vi "Test Type Selection.vi"(0 "File Path Control":path, 11 "Error In":errorcluster) -> (3 "path":path, 4 "File Name":string, 6 "Test Type":string, 8 "Interruptions":u32, 10 "Delay":u32, 15 "Error Out":errorcluster)   [LabVIEW 2018, in "CollectionSupport.lvlib"]
uses:
  CollectionSupport.lvlib
  Controls/Mech-Labial Test Types.ctl
panel:
  in  "Sex":u16(ring) items=["Male", "Female"]
  in  "Age":string
  in  "OK Button":bool
  in  "Subject":string
  in  "Test Types":T1 items=["Practice Trials", "Mechanical (Mask)", "Mechanical (Mouthpiece)", "Labial (Normal)", "Labial (Quiet)"]
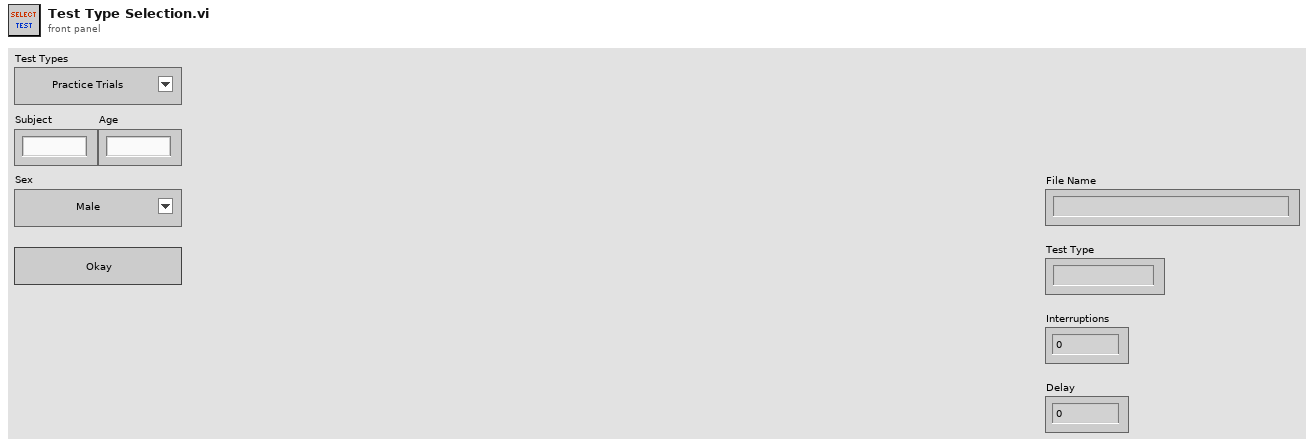
[diagram p1: front panel]
types:
  T1 = typedef "CollectionSupport.lvlib/Mech-Labial Test Types.ctl" = u16
  T2 = enum16{"open", "replace", "create", "open or create", "replace or create", "replace or create with confirmation"}
  T3 = typedef "eventvkey.ctl" = enum16{"ASCII", "Enter", "Return", "Shift", "Ctrl", "Alt", "Cmd", "Opt", "Caps", "NumLock", "Clear", "Break", "Up", "Down", "Left", "Right", "Insert", "Delete", "Home", "End", "PageUp", "PageDown", "Escape", "Help", "Pause", "ScrollLock", "F1", "F2", "F3", "F4", "F5", "F6", "F7", "F8", "F9", "F10", "F11", "F12", "F13", "F14", "F15", "F16", "F17", "F18", "F19", "F20", "F21", "F22", "F23", "F24", "Play", "VolumeUp", "VolumeDown", "Mute", "Two Byte Char"}
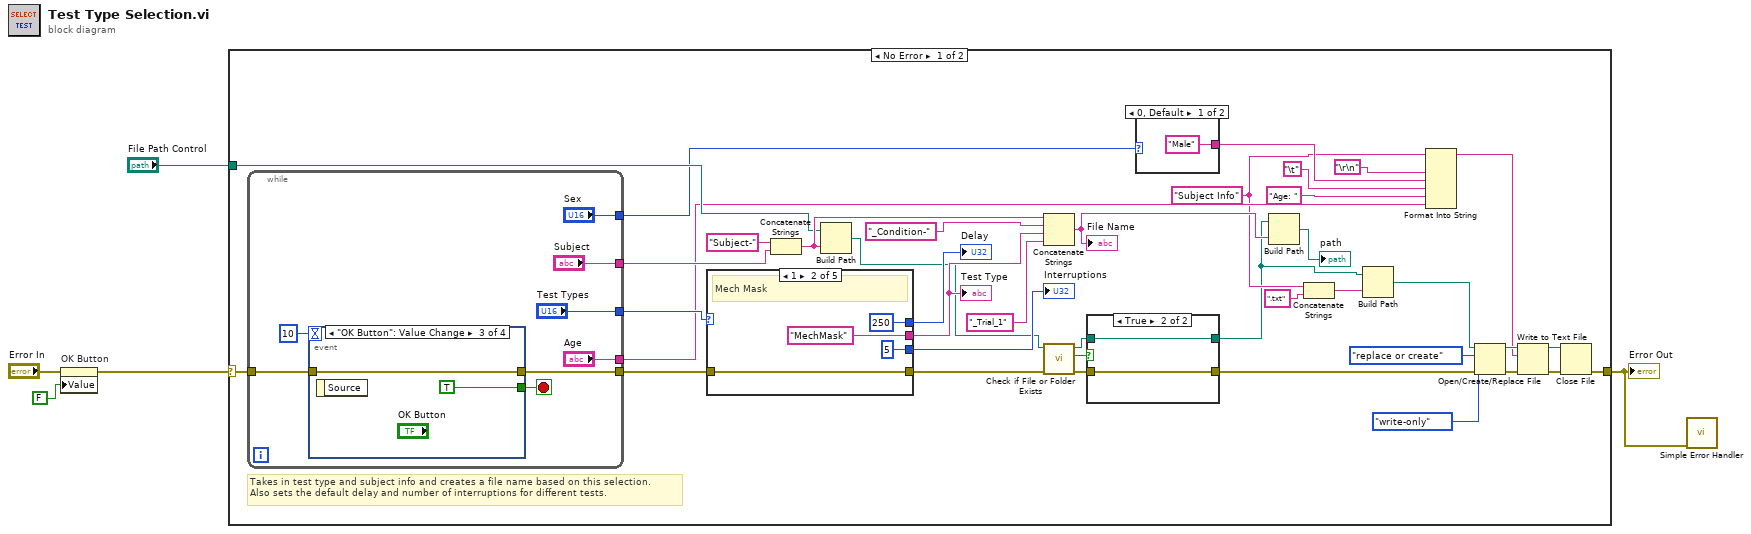
[diagram p0: block diagram]
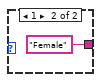
[diagram p2: hidden frame]
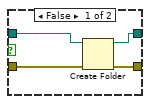
[diagram p3: hidden frame]
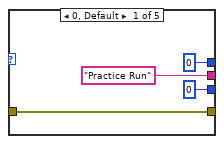
[diagram p4: hidden frame]
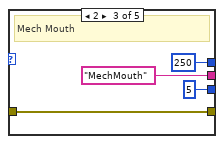
[diagram p5: hidden frame]
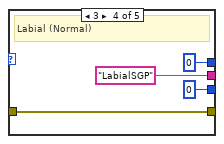
[diagram p6: hidden frame]
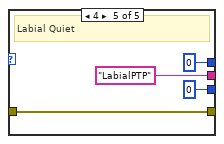
[diagram p7: hidden frame]
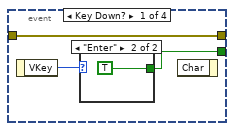
[diagram p8: hidden frame]
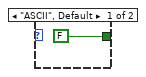
[diagram p9: hidden frame]
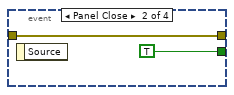
[diagram p10: hidden frame]
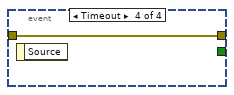
[diagram p11: hidden frame]
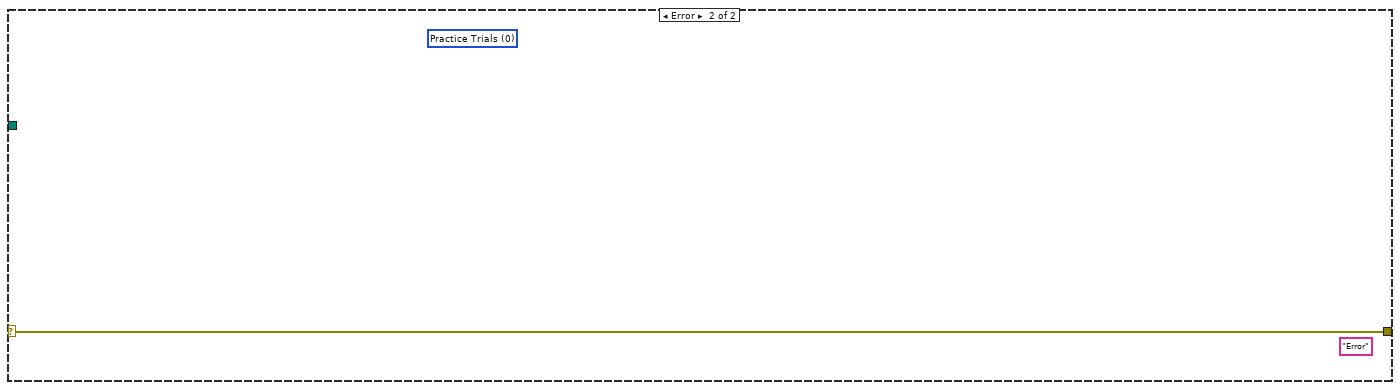
[diagram p12: hidden frame]
diagram:
  n1 = property on="OK Button" class="Bool (strict)"(error in="Error In", "Value"=FALSE ("Value (Signaling)")) -> (error out=w4:errorcluster)  [unwired: 1 in, 1 out]
  n2 = case shown="No Error" w4 {
    selector: w4 -> [w44 w91]
    tunnel: [w20 w91] -> w1
    tunnel: "File Path Control" -> [w28 _]
    frame No Error {
      w11 = "Subject Info" ("initial string")
      # "Takes in test type and subject info and creates a file name based on this selection. \nAlso sets the default delay and number of interruptions for different tests."
      n3 = while {
        tunnel: [w76] -> w38
        tunnel: w44 -> [w77]
        tunnel: ["Test Types"] -> w37
        tunnel: ["Subject"] -> w27
        tunnel: ["Sex"] -> w17
        tunnel: ["Age"] -> w13
        stop <- w80 stop-if-true
        n4 = event shown="[2] \"OK Button\": Value Change" {
          selector: _ -> [_ _ _ _]
          dyn-events: _ -> [_ _ _ _]
          timeout: 10 -> [_ _ _ _]
          tunnel: [w82 TRUE ("Value (Signaling)") TRUE _] -> w80
          tunnel: [w81 w86 w88 w90] -> w76
          tunnel: w77 -> [w81 w86 w88 w90]
          event Key Down? {
            n5 = event-data() -> ("VKey"=w83:T3)  [unwired: 1 in]
            n6 = case shown="\"Enter\"" w83 {
              tunnel: [FALSE ("Value (Signaling)") TRUE ("Value (Signaling)")] -> w82
              frame "ASCII", Default {
              }
              frame "Enter" {
              }
            }
            n7 = event-data() -> ()  [unwired: 2 in, 1 out]
          }
          event Panel Close {
            n8 = event-data() -> ()  [unwired: 1 in, 1 out]
          }
          event "OK Button": Value Change {
            n9 = event-data() -> ()  [unwired: 1 in, 1 out]
          }
          event Timeout {
            n10 = event-data() -> ()  [unwired: 1 in, 1 out]
          }
        }
      }
      n11 = case shown="1" w37 {
        tunnel: ["Practice Run" ("string") "MechMask" ("string") "MechMouth" ("string") "LabialSGP" ("string") "LabialPTP" ("string")] -> w43
        tunnel: [u32 0 ("Delay") u32 250 ("Delay") u32 250 ("Delay") u32 0 ("Delay") u32 0 ("Delay")] -> w40
        tunnel: [u32 0 ("Delay") u32 5 ("Delay") u32 5 ("Delay") u32 0 ("Delay") u32 0 ("Delay")] -> w39
        tunnel: w38 -> [w54 w57 w61 w65 w69]
        tunnel: [w54 w57 w61 w65 w69] -> w36
        frame 0, Default {
        }
        frame 1 {
          # "Mech Mask"
        }
        frame 2 {
          # "Mech Mouth"
        }
        frame 3 {
          # "Labial (Normal)"
        }
        frame 4 {
          # "Labial Quiet"
        }
      }
      "Interruptions" <- w39
      "Delay" <- w40
      "Test Type" <- w43
      n12 = Concatenate Strings("Subject-" ("default name"), w27) -> (w33:string)
      n13 = Build Path(base path=w28, name or relative path=w33) -> (appended path=w32:path)
      n14 = Concatenate Strings(w33, "_Condition-" ("string"), w43, "_Trial_1" ("string")) -> (w29:string)
      "File Name" <- w29
      n15 = call <vilib>:"Check if File or Folder Exists.vi"("error in (no error)"=w36, "path"=w32) -> ("error out"=w34:errorcluster, "file or folder exists?"=w35:bool, "dup path"=w31:path)  [unwired: 7 in]
      n16 = case shown="True" w35 {
        tunnel: w34 -> [w50 w52]
        tunnel: [w49 w52] -> w21
        tunnel: w31 -> [w48 w51]
        tunnel: [w47 w51] -> w7
        frame False {
          n17 = Create Folder(path (use dialog)=w48, error in=w50) -> (created path=w47:path, error out=w49:errorcluster)  [unwired: 1 in, 1 out]
        }
        frame True {
        }
      }
      n18 = case shown="0, Default" w17 {
        tunnel: ["Male" "Female"] -> w16
        frame 0, Default {
        }
        frame 1 {
        }
      }
      n19 = Build Path(base path=w7, name or relative path=w29) -> (appended path=→"path":path)
      n20 = Concatenate Strings(w11, ".txt" ("string")) -> (w9:string)
      n21 = Build Path(base path=w7, name or relative path=w9) -> (appended path=w18:path)
      n22 = Format Into String(initial string=w11, "\r\n", w16, "\t", "Age: " ("input 3"), w13) -> (resulting string=w12:string)  [unwired: 2 in, 1 out]
      n23 = Open/Create/Replace File(file path (use dialog)=w18, error in=w21, operation (0:open)=T2."replace or create", access (0:read/write)=enum16{"read/write", "read-only", "write-only"}."write-only") -> (refnum out=w23:refnum<file>, error out=w26:errorcluster)  [unwired: 2 in, 1 out]
      n24 = Write to Text File(file (use dialog)=w23, text=w12, error in=w26) -> (refnum out=w24:refnum<file>, error out=w25:errorcluster)  [unwired: 1 in, 1 out]
      n25 = Close File(refnum=w24, error in=w25) -> (error out=w20:errorcluster)  [unwired: 1 out]
    }
    frame Error {
      (unwired) "Error" ("Subject")
      (unwired) T1 0 items=["Practice Trials", "Mechanical (Mask)", "Mechanical (Mouthpiece)", "Labial (Normal)", "Labial (Quiet)"] ("Test Types")
    }
  }
  "Error Out" <- w1
  n26 = call <vilib>:"Simple Error Handler.vi"("error in (no error)"=w1) -> ()  [unwired: 4 in, 5 out]
